vi "Drive Controller.vi"(8 "error in":errorcluster) -> ()   [LabVIEW 2015]
doc: "This VI executes continuously carrying out the current operation and responding to updates or new operation requests. It will often contain the timing or control code that is difficult to place directly in TeleOp. This VI generally opens all sensors and motors and isolates the rest of the robot code from knowing implementation details of how the operations are carried out."
uses:
  <vilib>/Rock Robotics/WPI/CAN/TalonSRX/WPI_CANTalonSRX_GlobalStatus.ctl
  Drive Setpoints.ctl
  Drive Operations.ctl
  <vilib>/Rock Robotics/WPI/CAN/TalonSRX/WPI_CANTalonSRX_APIControlMode.ctl
  <vilib>/Rock Robotics/WPI/MotorControl/WPI_MotorControlOpenCANTalonSRX.vi
panel:
  out "Talon SRX Status":T1
  in  "Go":bool
  out "Out":dbl(knob) scale=-180.0..180.0
  in  "In":dbl(knob) scale=-180.0..180.0
  in  "Ramp Rate":dbl
  in  "I Zone":dbl
  in  "Apply":bool
  in  "F":dbl
  in  "D":dbl
  in  "I":dbl
  in  "P":dbl
  out "Setpoints":T2(graph)
  out "Current\nCmd":string
  # "Tip: It may be helpful to observe inputs and sensor values.\nYou may also want to display tuning or debugging controls."
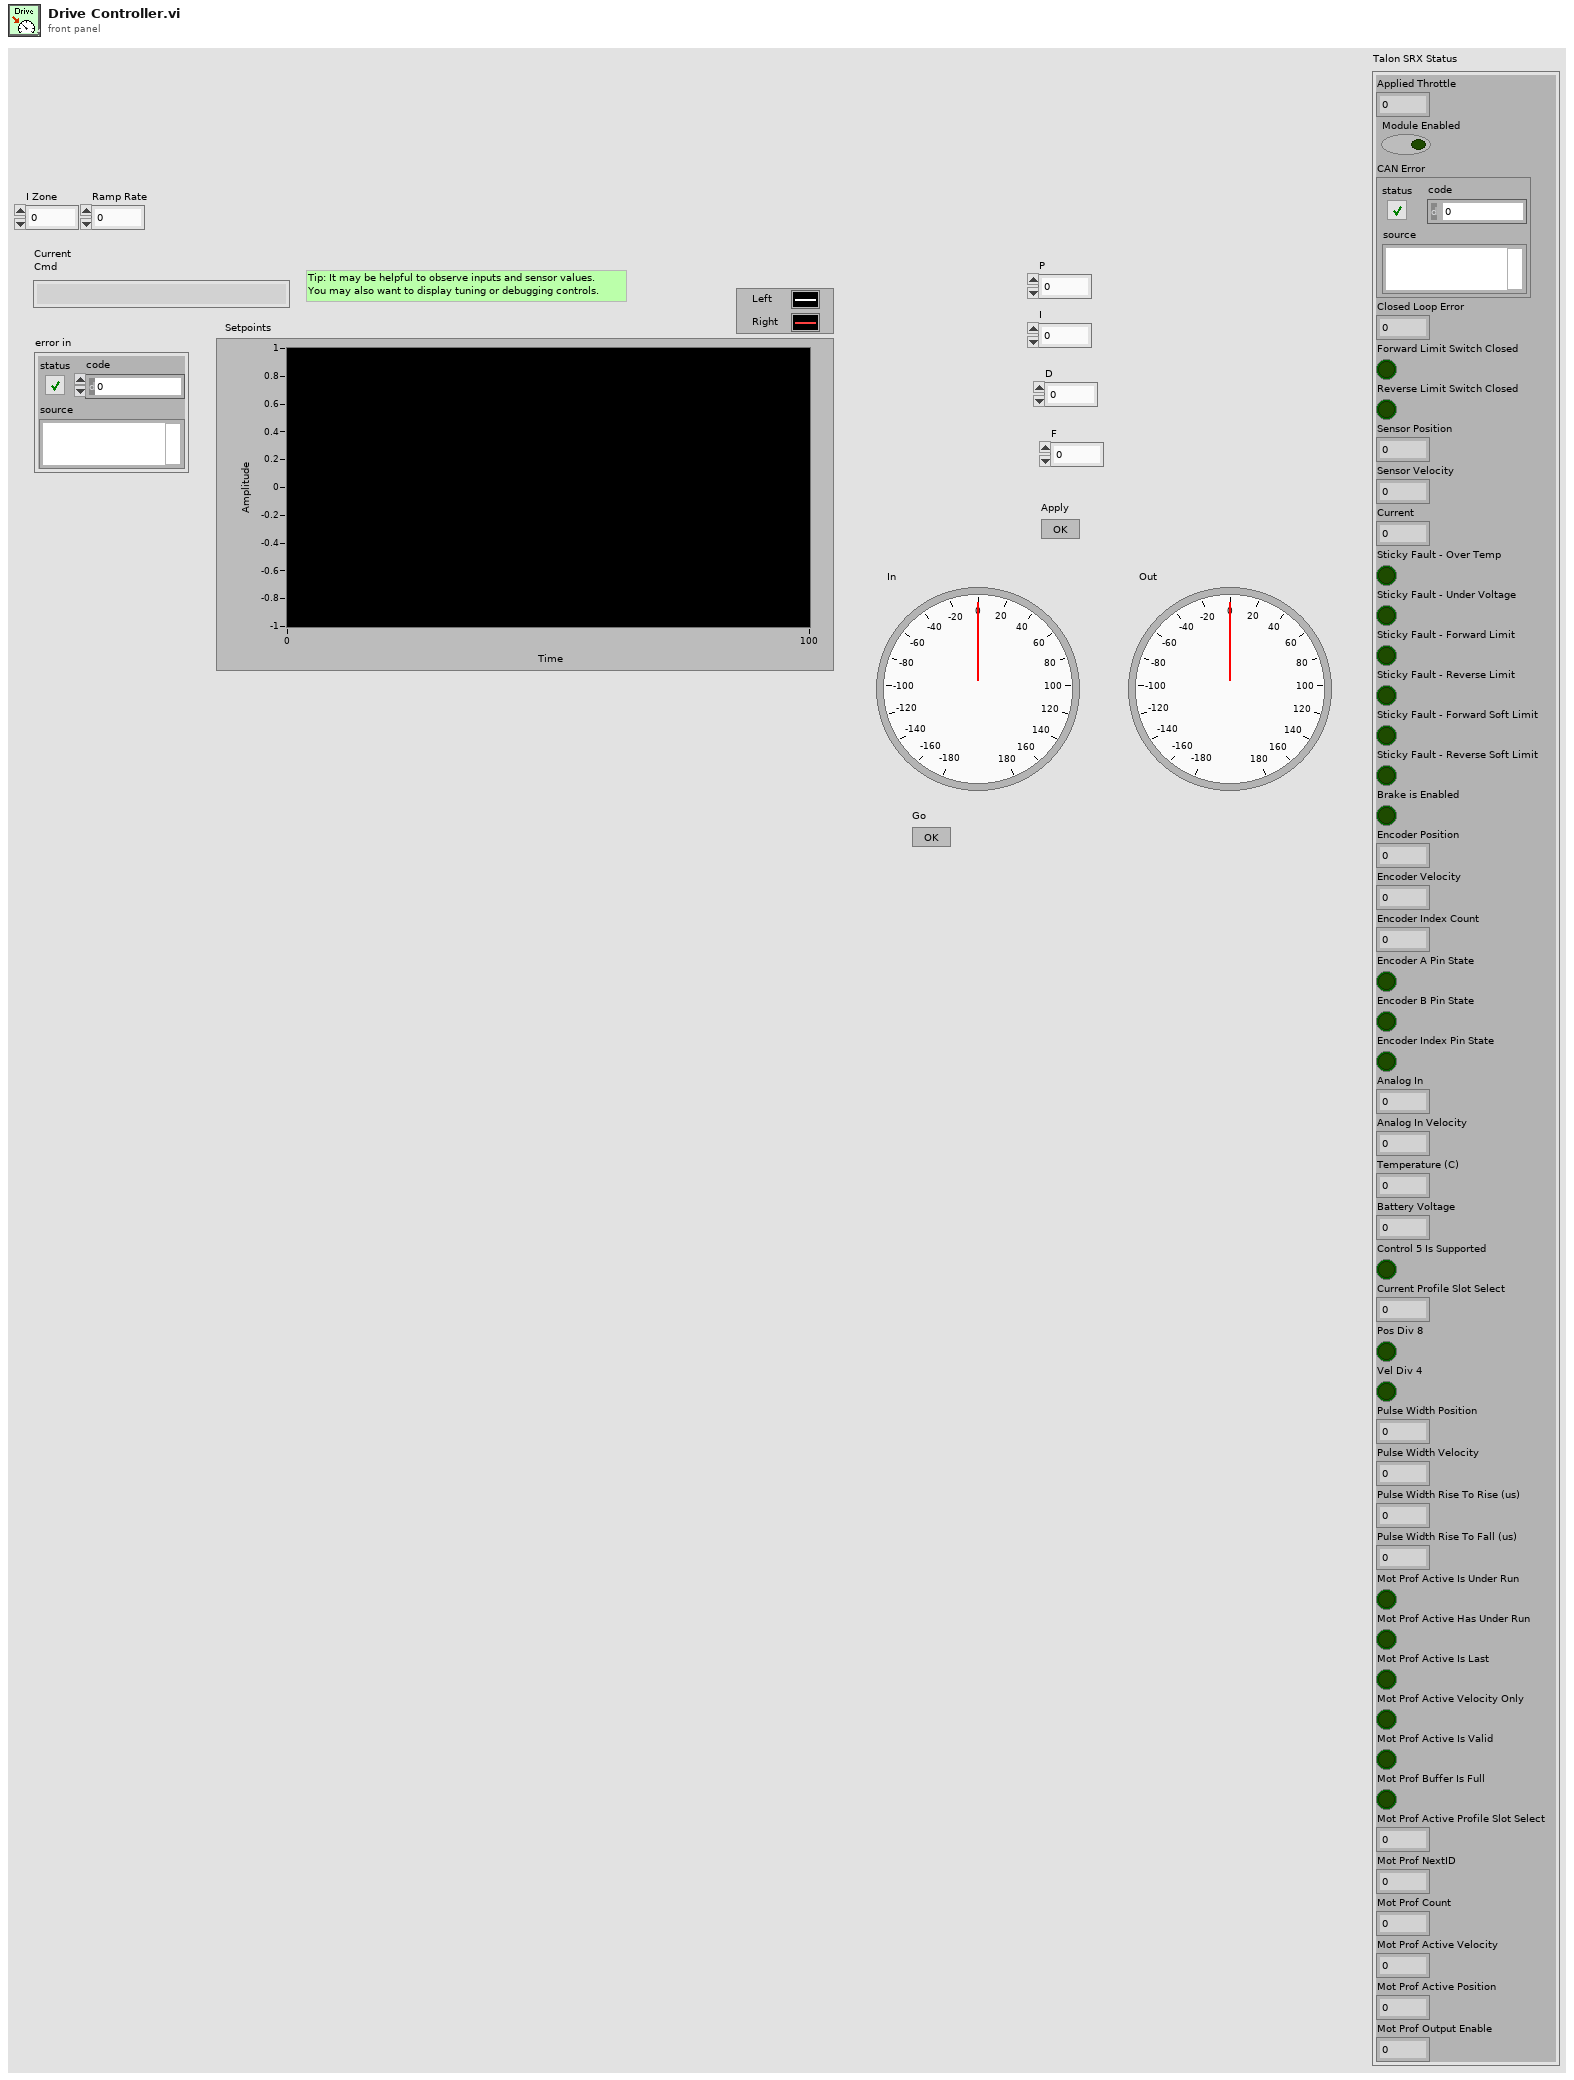
[diagram p1: front panel]
types:
  T1 = typedef "WPI_CANTalonSRX_GlobalStatus.ctl" = cluster{"Applied Throttle":dbl, "Module Enabled":bool, "CAN Error":errorcluster, "Closed Loop Error":dbl, "Forward Limit Switch Closed":bool, "Reverse Limit Switch Closed":bool, "Sensor Position":dbl, "Sensor Velocity":dbl, "Current":dbl, "Sticky Fault - Over Temp":bool, "Sticky Fault - Under Voltage":bool, "Sticky Fault - Forward Limit":bool, "Sticky Fault - Reverse Limit":bool, "Sticky Fault - Forward Soft Limit":bool, "Sticky Fault - Reverse Soft Limit":bool, "Brake is Enabled":bool, "Encoder Position":dbl, "Encoder Velocity":dbl, "Encoder Index Count":dbl, "Encoder A Pin State":bool, "Encoder B Pin State":bool, "Encoder Index Pin State":bool, "Analog In":dbl, "Analog In Velocity":dbl, "Temperature (C)":dbl, "Battery Voltage":dbl, "Control 5 Is Supported":bool, "Current Profile Slot Select":dbl, "Pos Div 8":bool, "Vel Div 4":bool, "Pulse Width Position":i32, "Pulse Width Velocity":i32, "Pulse Width Rise To Rise (us)":i32, "Pulse Width Rise To Fall (us)":i32, "Mot Prof Active Is Under Run":bool, "Mot Prof Active Has Under Run":bool, "Mot Prof Active Is Last":bool, "Mot Prof Active Velocity Only":bool, "Mot Prof Active Is Valid":bool, "Mot Prof Buffer Is Full":bool, "Mot Prof Active Profile Slot Select":i32, "Mot Prof NextID":i32, "Mot Prof Count":i32, "Mot Prof Active Velocity":dbl, "Mot Prof Active Position":dbl, "Mot Prof Output Enable":i32}
  T2 = cluster{"Left Setpoint":dbl, "Right Setpoint":dbl}
  T3 = typedef "WPI_CANTalonSRX_APIControlMode.ctl" = enum8{"Percent VBus", "Speed", "Position", "Slave", "Unchanged / Invalid", "Voltage Compensation", "Current", "Motion Profile"}
  T4 = typedef "Drive Setpoints.ctl" = cluster{"Operation":T5, "Left Setpoint":dbl, "Right Setpoint":dbl, "Duration":dbl}
  T5 = typedef "Drive Operations.ctl" = enum16{"Reserve", "Read Current", "Immediate", "Drive for Time", "Drive for Distance"}
  T6 = typedef "WPI_MotorControlDeviceRef.ctl" = cluster{"DeviceStatus":errorcluster, "Type":T7, "PWM":cluster{"PWM Channel":T8, "DeadBand":T9}, "CAN":cluster{"Device Number":u8, "Control Mode":T10, "Semaphore":T11, "Max Vout":dbl, "TalonSRX Control Mode":T3}, "Invert":bool}
  T7 = typedef "WPI_MotorControlType.ctl" = enum16{"PWM", "CAN", "CANTalonSRX"}
  T8 = typedef "FPGA_DIOPWMChannel.ctl" = enum8{"PWM 0", "PWM 1", "PWM 2", "PWM 3", "PWM 4", "PWM 5", "PWM 6", "PWM 7", "PWM 8", "PWM 9", "PWM MXP 0", "PWM MXP 1", "PWM MXP 2", "PWM MXP 3", "PWM MXP 4", "PWM MXP 5", "PWM MXP 6", "PWM MXP 7", "PWM MXP 8", "PWM MXP 9", "Invalid"}
  T9 = typedef "WPI_PWMDeadband.ctl" = cluster{"Name":string, "maxPositivePwm":i32, "minPositivePwm":i32, "centerPwm":i32, "maxNegativePwm":i32, "minNegativePwm":i32, "angularRange":u16}
  T10 = typedef "WPI_CANJaguar_ControlMode.ctl" = enum8{"Percent VBus", "Current", "Speed", "Position", "Voltage"}
  T11 = typedef "Semaphore RefNum" = refnum<k1>
  T12 = typedef "Command Status Info.ctl" = cluster{"Name":string, "Status":T13, "notifier out":T14}
  T13 = typedef "Completion Status.ctl" = enum16{"Successful", "Aborted", "Incomplete"}
  T14 = typedef "Completion Notifier.ctl" = refnum<notifier>
  T15 = cluster{"SubSystem Data":T4, cluster{"Start Time (ms)":u32, "Iterations":i32}, cluster{"Command Info":T12, "Description":string, "SubSystem Data":T4, "notifier out":refnum<notifier>, "Subsystem Name":string}}
  T16 = cluster{"SubSystem Data":T4, cluster{"Start Time (ms)":u32, "Iterations":i32}, "Default Command Arguments":cluster{"Command Info":T12, "Description":string, "SubSystem Data":T4, "notifier out":refnum<notifier>, "Subsystem Name":string}}
  T17 = cluster{"Don't move motors while reserved":dbl, "Don't move motors while reserved":dbl}
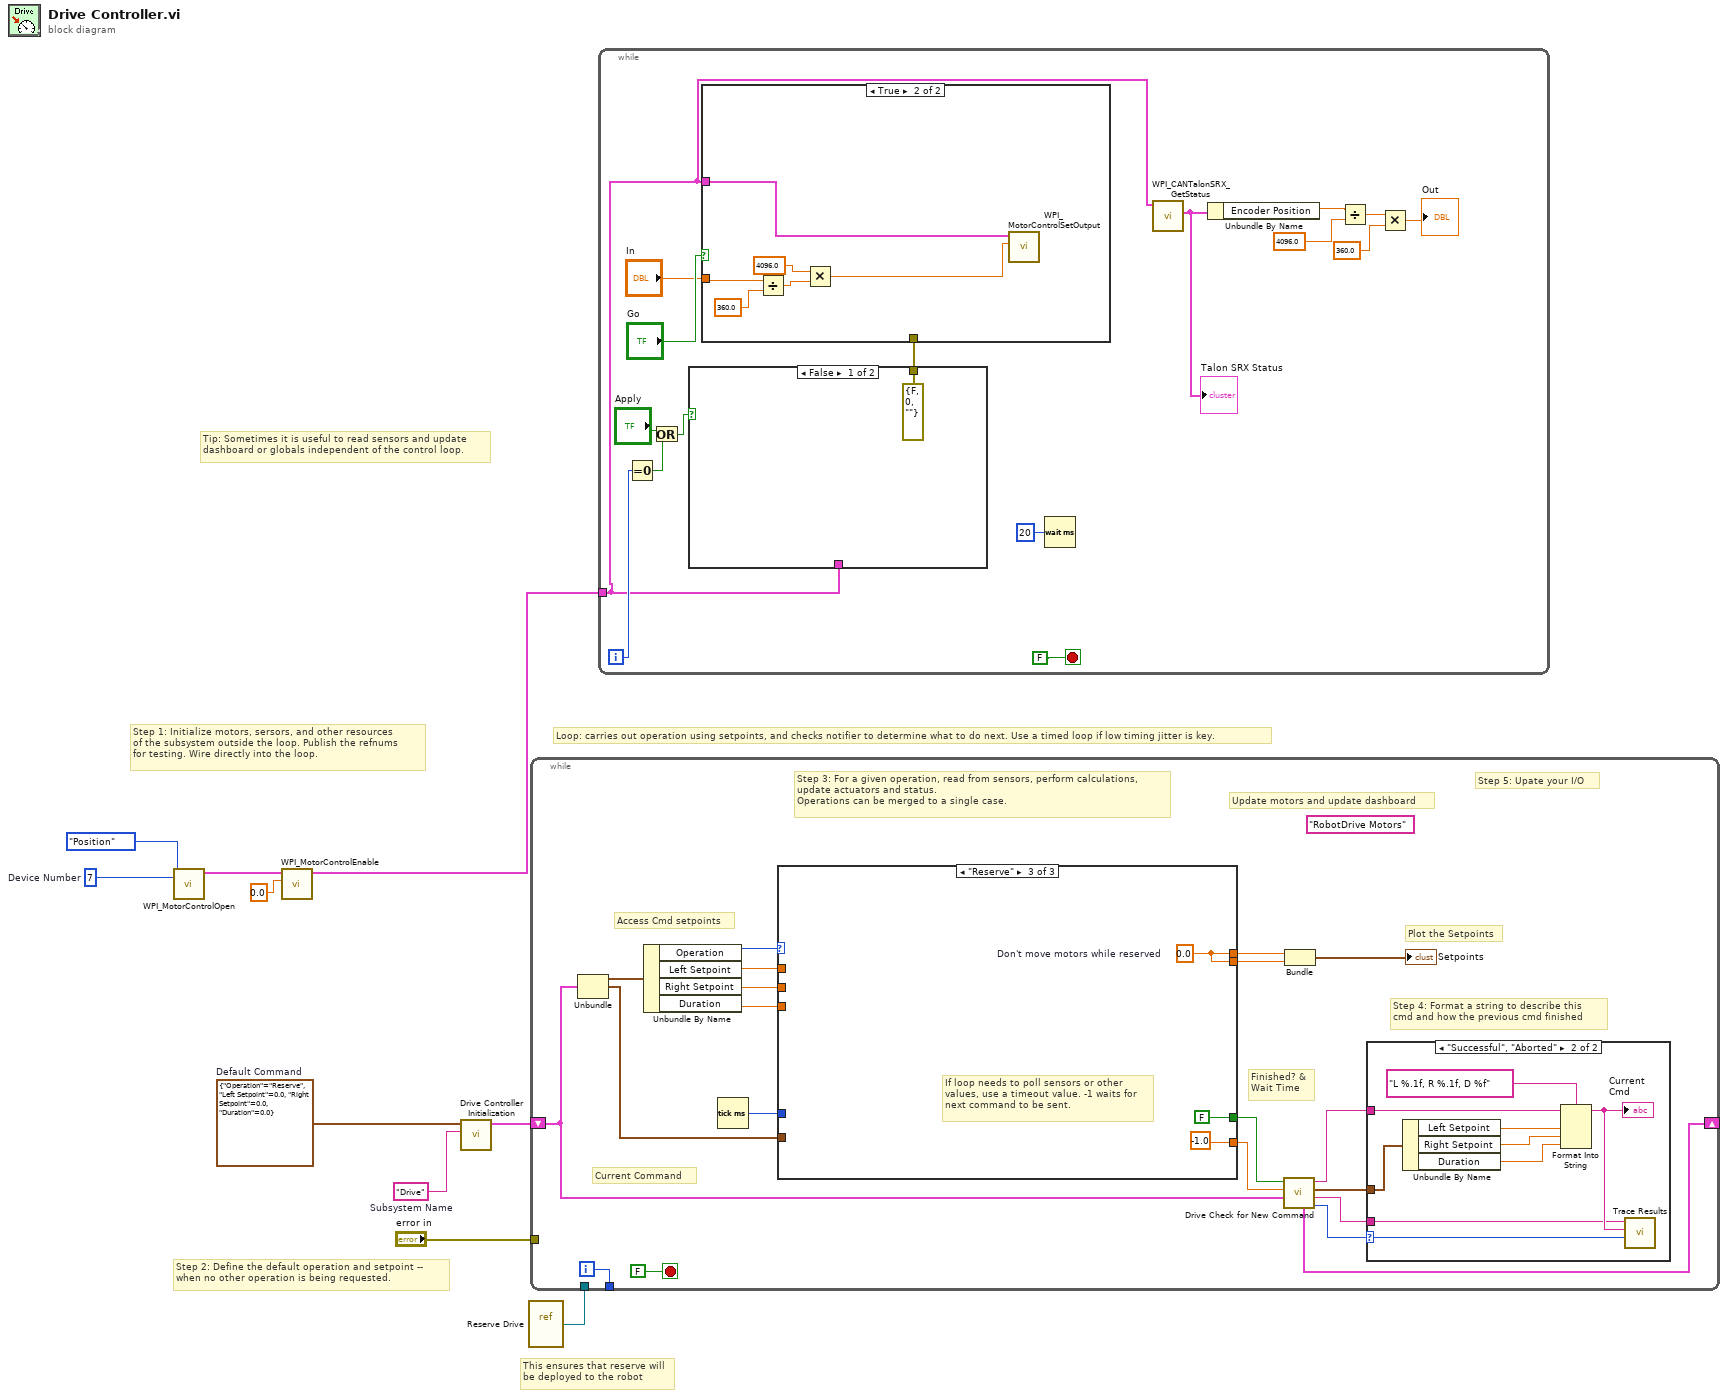
[diagram p0: block diagram]
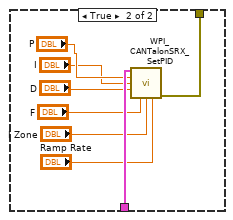
[diagram p3: hidden frame]
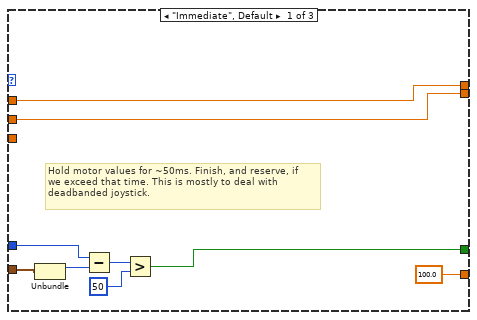
[diagram p5: hidden frame]
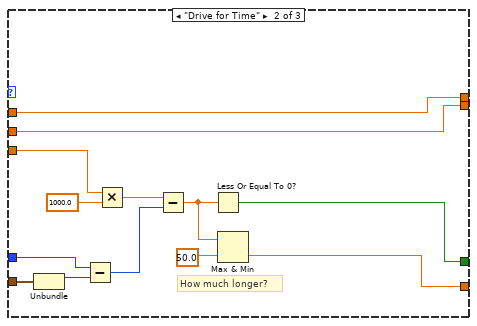
[diagram p6: hidden frame]
diagram:
  w4 = u8 7  # Device Number
  w9 = T4 {"Operation"=enum."Reserve", "Left Setpoint"=0.0, "Right Setpoint"=0.0, "Duration"=0.0}  # Default Command
  w10 = "Drive"  # Subsystem Name
  # "This ensures that reserve will\nbe deployed to the robot"
  # "Tip: Sometimes it is useful to read sensors and update\ndashboard or globals independent of the control loop."
  # "Step 2: Define the default operation and setpoint --\nwhen no other operation is being requested."
  # "Step 1: Initialize motors, sersors, and other resources\nof the subsystem outside the loop. Publish the refnums\nfor testing. Wire directly into the loop."
  # "Loop: carries out operation using setpoints, and checks notifier to determine what to do next. Use a timed loop if low timing jitter is key."
  n1 = call-poly <vilib>:"WPI_MotorControlOpen.vi"("Device Number"=w4, "Control Mode"=WPI_CANTalonSRX_APIControlMode."Position") -> ("MotorControlDeviceRef"=w3:T6)  [unwired: 8 in, 1 out]
  n2 = call <vilib>:"WPI_MotorControlEnable.vi"("Encoder Initial Position"=0.0, "CAN MotorDevRef"=w3) -> ("CAN MotorDevRef"=w2:T6)  [unwired: 8 in, 1 out]
  n3 = call "Drive Controller Initialization.vi"("Subsystem Name"=w10, "Default Command"=w9) -> ("output cluster"=w7:T15)  [unwired: 9 in]
  n4 = vi-ref "Reserve Drive.vi"() -> (w6:refnum<vi>)
  n5 = while {
    shift-right: [w18] -> _
    shift-left: w7 -> [w11]
    tunnel: [w29] -> _
    tunnel: "error in" -> [_]
    tunnel: w6 -> [_]
    i -> [w29]
    stop <- FALSE stop-if-true
    (unwired) "RobotDrive Motors" ("Name")
    # "Step 5: Upate your I/O"
    # "Step 4: Format a string to describe this\ncmd and how the previous cmd finished"
    # "Current Command"
    # "Update motors and update dashboard"
    # "Plot the Setpoints"
    # "Access Cmd setpoints"
    # "Finished? &\nWait Time"
    # "Step 3: For a given operation, read from sensors, perform calculations,\nupdate actuators and status.\nOperations can be merged to a single case."
    n6 = Unbundle(w11) -> ("SubSystem Data"=w25:T4, w12:cluster{"Start Time (ms)":u32, "Iterations":i32})  [unwired: 1 out]
    n7 = Unbundle By Name(w25) -> ("Operation"=w24:T5, "Left Setpoint"=w23:dbl, "Right Setpoint"=w22:dbl, "Duration"=w21:dbl)
    n8 = Tick Count (ms)() -> (millisecond timer value=w20:u32)
    n9 = case shown="\"Reserve\"" w24 {
      tunnel: [100.0 w49 -1.0] -> w17
      tunnel: [w41 w56 FALSE ("ignore previous (F)")] -> w16
      tunnel: w12 -> [w40 w58 _]
      tunnel: [w47 w55 w62] -> w27
      tunnel: [w46 w54 w62] -> w26
      tunnel: w23 -> [w47 w55 _]
      tunnel: w22 -> [w46 w54 _]
      tunnel: w21 -> [_ w53 _]
      tunnel: w20 -> [w42 w52 _]
      frame "Immediate", Default {
        # "Hold motor values for ~50ms. Finish, and reserve, if\nwe exceed that time. This is mostly to deal with\ndeadbanded joystick."
        n10 = Unbundle(w40) -> ("Start Time (ms)"=w43:u32)  [unwired: 1 out]
        n11 = Subtract(x=w42, y=w43) -> (x-y=w44:u32)
        n12 = Greater?(x=w44, y=u8 50 ("Left Motor")) -> (0:w41:bool)
      }
      frame "Drive for Time" {
        # "How much longer?"
        n13 = Unbundle(w58) -> ("Start Time (ms)"=w57:u32)  [unwired: 1 out]
        n14 = Subtract(x=w52, y=w57) -> (x-y=w61:u32)
        n15 = Multiply(x=w53, y=1000.0) -> (x*y=w60:dbl)
        n16 = Subtract(x=w60, y=w61) -> (x-y=w51:dbl)
        n17 = Less Or Equal To 0?(x=w51) -> (x <= 0?=w56:bool)
        n18 = Max & Min(x=w51, y=50.0) -> (min(x,y)=w49:dbl)  [unwired: 1 out]
      }
      frame "Reserve" {
        w62 = 0.0  # Don't move motors while reserved
        # "If loop needs to poll sensors or other\nvalues, use a timeout value. -1 waits for\nnext command to be sent."
      }
    }
    n19 = call "Drive Check for New Command.vi"("input cluster"=w11, "Wait time (ms)"=w17, "Finished?"=w16) -> ("Completion"=w19:T13, "Subsystem Name"=w13:string, "SetPoint"=w14:T4, "Initial Trace String"=w15:string, "output cluster"=w18:T16)  [unwired: 4 in]
    n20 = Bundle("Don't move motors while reserved"=w27, "Don't move motors while reserved"=w26) -> (→"Setpoints":T17)  [unwired: 1 in]
    n21 = case shown="\"Successful\", \"Aborted\"" w19 {
      selector: w19 -> [_ w39]
      tunnel: w15 -> [_ w34]
      tunnel: w14 -> [_ w35]
      tunnel: w13 -> [_ w31]
      frame "Incomplete", Default {
        # "Continuing current command"
      }
      frame "Successful", "Aborted" {
        # "Report and setup for next command"
        n22 = Unbundle By Name(w35) -> ("Left Setpoint"=w37:dbl, "Right Setpoint"=w38:dbl, "Duration"=w32:dbl)
        n23 = Format Into String(format string="L %.1f, R %.1f, D %f", initial string=w34, w37, w38, w32) -> (resulting string=w33:string)  [unwired: 1 in, 1 out]
        "Current\nCmd" <- w33
        n24 = call <vilib>:"Trace Results.vi"("Status of previous command"=w39, "Description"=w33, "Subsystem"=w31) -> ()  [unwired: 9 in]
      }
    }
  }
  n25 = while {
    tunnel: w2 -> [w71]
    i -> [w75]
    stop <- FALSE stop-if-true
    n26 = Equal To 0?(x=w75) -> (x = 0?=w76:bool)
    n27 = Or(x="Apply", y=w76) -> (x .or. y?=w77:bool)
    n28 = case shown="False" w77 {
      tunnel: w71 -> [_ w95]
      tunnel: [errorcluster {"status"=FALSE, "code"=0, "source"=""} ("error out") w88] -> w72
      frame False {
      }
      frame True {
        n29 = call <vilib>:"WPI_CANTalonSRX_SetPID.vi"("CAN Talon SRX Ref"=w95, "P"="P", "I"="I", "D"="D", "F"="F", "I Zone"="I Zone", "Ramp Rate"="Ramp Rate") -> ("error out"=w88:errorcluster)  [unwired: 7 in, 1 out]
      }
    }
    n30 = case shown="True" "Go" {
      tunnel: "In" -> [_ w85]
      tunnel: w71 -> [_ w86]
      tunnel: w72 -> [_ _]
      frame False {
      }
      frame True {
        n31 = Divide(x=w85, y=360.0) -> (x/y=w83:dbl)
        n32 = Multiply(x=4096.0, y=w83) -> (x*y=w81:dbl)
        n33 = call <vilib>:"WPI_MotorControlSetOutput.vi"("Output"=w81, "MotorControlDevRef"=w86) -> ()  [unwired: 7 in, 3 out]
      }
    }
    n34 = Wait (ms)(milliseconds to wait=u32 20) -> ()  [unwired: 1 out]
    n35 = call <vilib>:"WPI_CANTalonSRX_GetStatus.vi"("CAN Talon SRX Ref"=w71) -> ("Talon SRX Status"=w70:T1)  [unwired: 8 in, 2 out]
    "Talon SRX Status" <- w70
    n36 = Unbundle By Name(w70) -> ("Encoder Position"=w67:dbl)
    n37 = Divide(x=w67, y=4096.0) -> (x/y=w65:dbl)
    n38 = Multiply(x=w65, y=360.0) -> (x*y=→"Out":dbl)
  }
